vi "Read exit.vi"(8 "error in (no error)":errorcluster, 11 "Communication Channel in":refnum<class "Communication Channel.lvclass">) -> (0 "error out":errorcluster, 2 "exit":bool, 3 "Communication Channel out":refnum<class "Communication Channel.lvclass">)   [LabVIEW 2018, in "Communication Channel.lvclass"]
uses:
  Communication Channel.lvclass
  Communication Channel.lvclass/Communication Channel.ctl
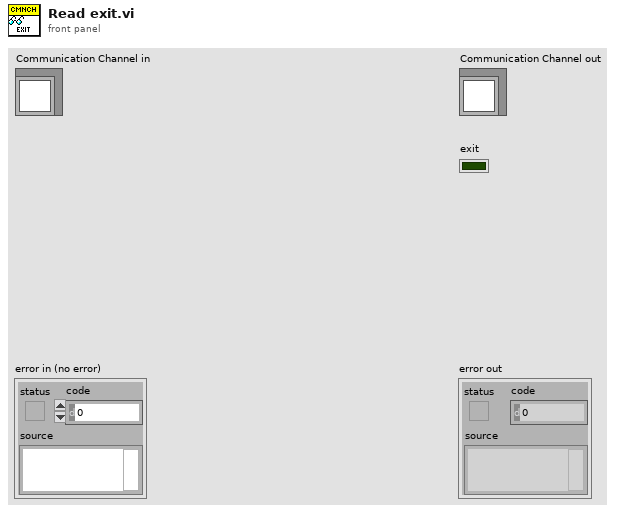
[diagram p1: front panel]
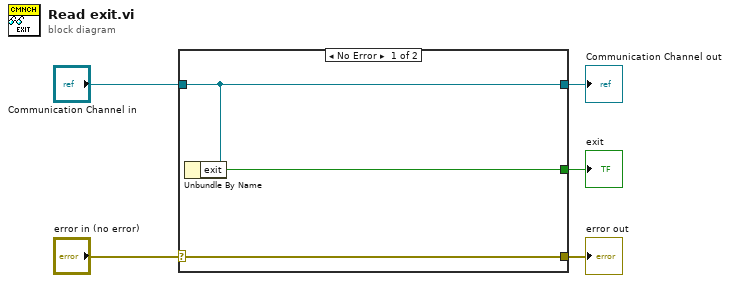
[diagram p0: block diagram]
diagram:
  n1 = case shown="No Error" "error in (no error)" {
    selector: "error in (no error)" -> [w8 w9]
    tunnel: [w8 w9] -> w4
    tunnel: [w7 w10] -> w2
    tunnel: "Communication Channel in" -> [w7 w10]
    tunnel: [w6 _] -> w1
    frame No Error {
      n2 = Unbundle By Name(w7) -> ("exit"=w6:bool)
    }
    frame Error {
    }
  }
  "error out" <- w4
  "Communication Channel out" <- w2
  "exit" <- w1
